vi "Test vi.vi"() -> ()   [LabVIEW 2020, in "FT-IR.lvlib" / "Get Spectra.lvlib"]
uses:
  Get Spectra.lvlib
  Grafik/Diagramm_NEU.ctl
  ReadLabFile/Spectrum FILE.ctl
  ReadLabFile/User arrays.ctl
  ReadLabFile/Sub spectra.ctl
  ReadLabFile/Spectrum.ctl
  ReadLabFile/Aktionen Lab File.ctl
  Aktion FGV Background-Daten.ctl
  ReadLabFile/Read Lab File.lvlib
  <vilib>/Waveform/WDTOps.llb/WDT Get Waveform Subset SGL.vi
  Grafik/Grafik.lvlib
panel:
  out "XY-Graph 4":cluster{dbl[], "Y":dbl[]}[](graph)
  out "Graph 2":T1
  out "XY-Graph 3":cluster{dbl[], "Y":dbl[]}(graph)
  out "Zeitstempel":timestamp
  out "DATE AND TIME":u32
  out "XY-Graph 2":cluster{dbl[], "[Y]":sgl[]}[](graph)
  out "XY-Graph":cluster{dbl[], "[Y]":sgl[]}[](graph)
  out "Signalverlaufsgraph":waveform(sgl)(graph)
  in  "Spectrum  FILE Name":path=path "C:/OLT/backgrnd.lab"
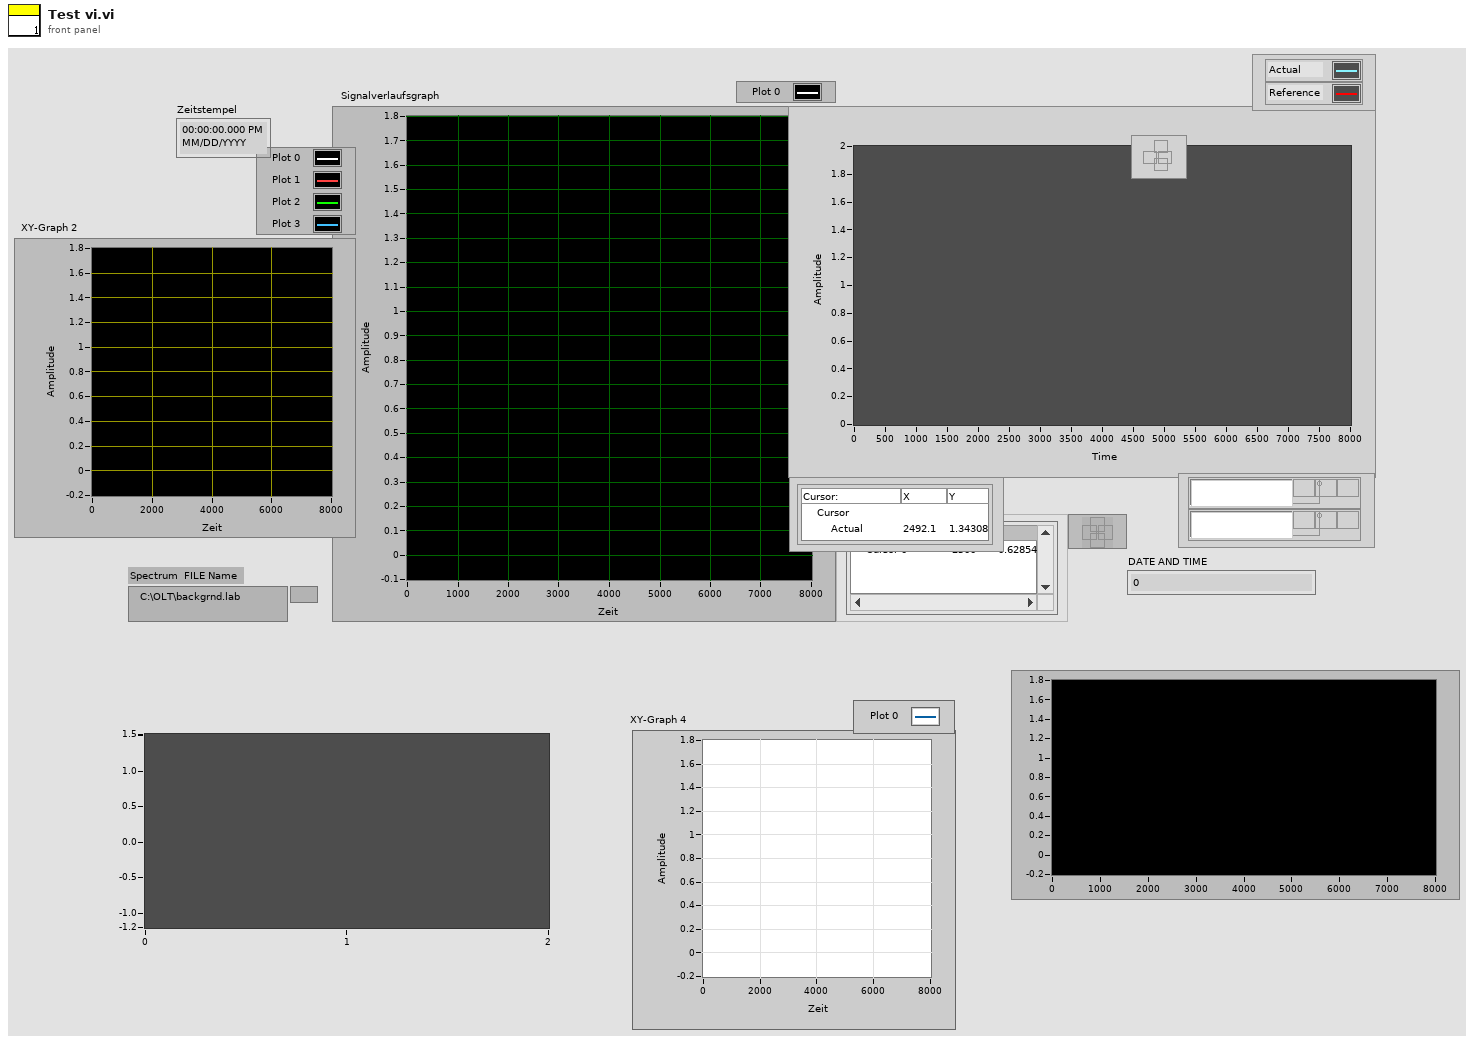
[diagram p1: front panel]
types:
  T1 = typedef "Grafik.lvlib/Diagramm_NEU.ctl" = waveform(dbl)
  T2 = typedef "FT-IR.lvlib/Get Spectra.lvlib/Aktion FGV Background-Daten.ctl" = enum16{"lesen", "schreiben", "Background aktiv", "Referenz", "laden", "speichern", "Plot sichtbar"}
  T3 = typedef "FT-IR.lvlib/Read Lab File.lvlib/Aktionen Lab File.ctl" = enum16{"lesen", "laden"}
  T4 = typedef "FT-IR.lvlib/Read Lab File.lvlib/Spectrum FILE.ctl" = cluster{"MEMO":string, "User arrays":T5, "SPECTRA":T6}
  T5 = typedef "FT-IR.lvlib/Read Lab File.lvlib/User arrays.ctl" = cluster{"Tag":string, "User double":dbl[]}[]
  T6 = typedef "FT-IR.lvlib/Read Lab File.lvlib/Sub spectra.ctl" = cluster{"Tag":string, "DATE AND TIME":u32, "spectrum":T7}[]
  T7 = typedef "FT-IR.lvlib/Read Lab File.lvlib/Spectrum.ctl" = cluster{"x0":dbl, "dx":dbl, "[Y]":sgl[]}
  T8 = cluster{"Tag":string, "DATE AND TIME":u32, "spectrum":T7}
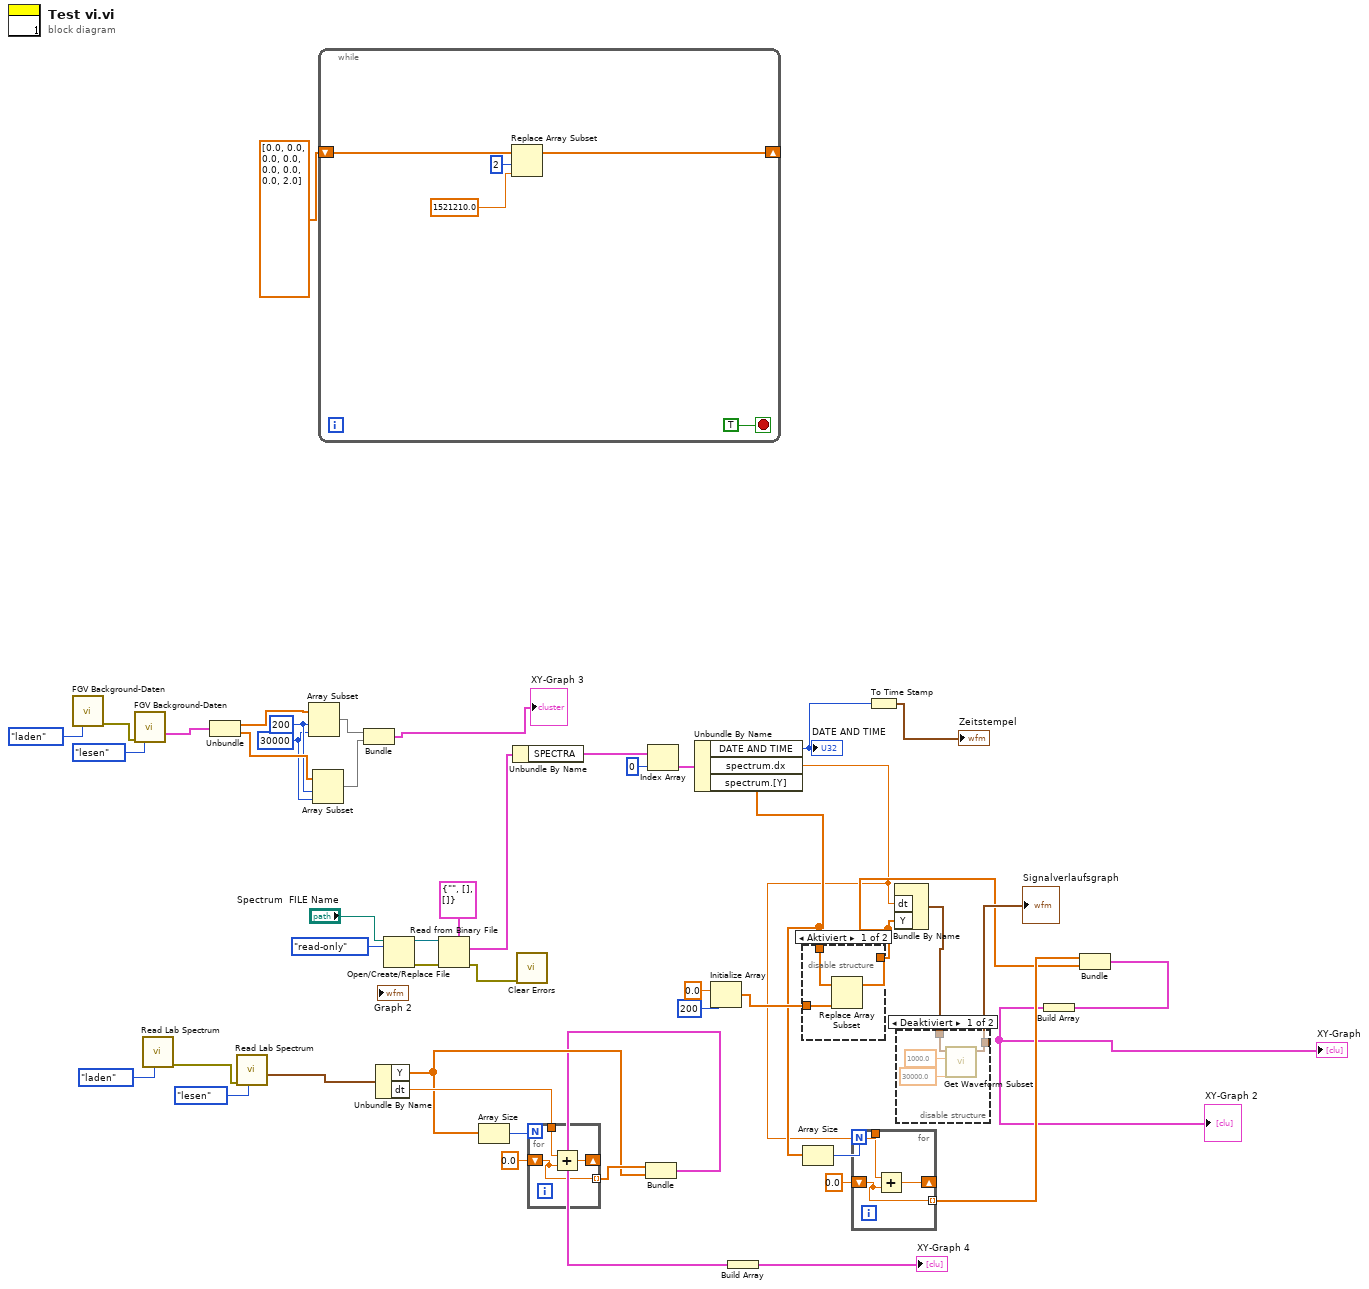
[diagram p0: block diagram]
diagram:
  w2 = 30000 ("Länge")
  w3 = 200 ("Index")
  n1 = call "FGV Background-Daten.vi"("Aktion"=Aktion_FGV_Background-Daten."laden") -> ("error out"=w12:errorcluster)  [unwired: 7 in, 7 out]
  n2 = call "FGV Background-Daten.vi"("error in (no error)"=w12, "Aktion"=Aktion_FGV_Background-Daten."lesen") -> ("Referenz"=w9:cluster{"Ramp Pattern":dbl[], dbl[]})  [unwired: 6 in, 7 out]
  n3 = call "Read Lab Spectrum.VI"("Aktionen"=Aktionen_Lab_File."laden") -> ("error out"=w22:errorcluster)  [unwired: 7 in, 3 out]
  n4 = Unbundle(w9) -> ("Ramp Pattern"=w8:dbl[], w7:dbl[])
  n5 = call "Read Lab Spectrum.VI"("Aktionen"=Aktionen_Lab_File."lesen", "error in (no error)"=w22) -> ("Graph 1"=w21:T1)  [unwired: 6 in, 3 out]
  n6 = Array Subset(array=w8, index=w3, length=w2) -> (w6:dbl[])
  n7 = Array Subset(array=w7, index=w3, length=w2) -> (w5:dbl[])
  n8 = while {
    shift-right: [w51] -> _
    shift-left: dbl[] [0.0, 0.0, 0.0, 0.0, 0.0, 0.0, 0.0, 2.0] -> [w50]
    stop <- TRUE stop-if-true
    n9 = Replace Array Subset(array=w50, new element=1521210.0, index=2 ("Index")) -> (w51:dbl[])
  }
  n10 = Bundle(w6, w5) -> (→"XY-Graph 3":cluster{dbl[], dbl[]})  [unwired: 1 in]
  n11 = Unbundle By Name(w21) -> ("Y"=w16:dbl[], "dt"=w18:dbl)
  n12 = Open/Create/Replace File(file path (use dialog)="Spectrum  FILE Name", access (0:read/write)=enum16{"read/write", "read-only", "write-only"}."read-only" ("Zugriff (0:Lesen/Schreiben)")) -> (refnum out=w44:refnum<file>, error out=w45:errorcluster)  [unwired: 1 in, 4 out]
  n13 = Read from Binary File(5:T4 {"MEMO"="", "User arrays"=[], "SPECTRA"=[]} ("empty Spectrum FILE"), 8:w45, 11:w44) -> (0:w27:errorcluster, 2:w41:T4)  [unwired: 5 out]
  n14 = Array Size(array=w16) -> (size(s)=w19:i32)
  n15 = Unbundle By Name(w41) -> ("SPECTRA"=w42:T6)
  n16 = call <vilib>:"Clear Errors.vi"("error in (no error)"=w27) -> ()  [unwired: 5 in, 2 out]
  n17 = for {
    N: w19 -> [_]
    tunnel: [w55] -> w17 mode=indexing
    shift-right: [w56] -> _
    shift-left: 0.0 -> [w55]
    tunnel: w18 -> [w54]
    n18 = Add(x=w54, y=w55) -> (x+y=w56:dbl)
  }
  n19 = Bundle(w17, "Y"=w16) -> (w15:cluster{dbl[], "Y":dbl[]})  [unwired: 1 in]
  n20 = Index Array(array=w42, index=0 ("Index")) -> (element=w43:T8)
  n21 = Unbundle By Name(w43) -> ("DATE AND TIME"=w26:u32, "spectrum.dx"=w10:dbl, "spectrum.[Y]"=w32:sgl[])
  "DATE AND TIME" <- w26
  n22 = Initialize Array(0.0 ("Element"), 200 ("Dimensionsgröße")) -> (w37:dbl[])
  n23 = Build Array(w15) -> (→"XY-Graph 4":cluster{dbl[], "Y":dbl[]}[])
  n24 = disable-structure shown="Aktiviert" {
    disable-tunnel: w32 -> [w59 w60]
    disable-tunnel: [w58 w60] -> w28
    disable-tunnel: w37 -> [w57 _]
    frame Enabled {
      n25 = Replace Array Subset(array=w59, new element=w57) -> (w58:sgl[])  [unwired: 1 in]
    }
    frame Disabled {
    }
  }
  n26 = Array Size(array=w32) -> (size(s)=w34:i32)
  n27 = for {
    N: w34 -> [_]
    tunnel: [w62] -> w33 mode=indexing
    shift-right: [w63] -> _
    shift-left: 0.0 -> [w62]
    tunnel: w10 -> [w61]
    n28 = Add(x=w61, y=w62) -> (x+y=w63:dbl)
  }
  n29 = To Time Stamp(1:w26) -> (0:→"Zeitstempel":timestamp)
  n30 = Bundle By Name("dt"=w10, "Y"=w28) -> (w36:waveform(sgl))  [unwired: 1 in]
  n31 = disable-structure shown="Deaktiviert" {
    disable-tunnel: w36 -> [w67 w68]
    disable-tunnel: [w66 w68] -> w35
    frame Disabled {
      n32 = call-poly <vilib>:"Get Waveform Subset.vi"("duration"=30000.0, "start samples/time"=1000.0, "waveform in"=w67) -> ("waveform out"=w66:waveform(sgl))  [unwired: 3 in, 3 out]
    }
    frame Enabled {
    }
  }
  "Signalverlaufsgraph" <- w35
  n33 = Bundle(w33, "[Y]"=w28) -> (w31:cluster{dbl[], "[Y]":sgl[]})  [unwired: 1 in]
  n34 = Build Array(w31) -> (→"XY-Graph" →"XY-Graph 2":cluster{dbl[], "[Y]":sgl[]}[])
